vi "Neighbour Status.vi"(0 "Cell":i32, 5 "Parsed Board":T1, 11 "error in (no error)":errorcluster) -> (4 "Full?":bool, 6 "Min Count to Max":i32, 8 "Cell Index":i32, 15 "error out":errorcluster)   [LabVIEW 2014]
uses:
  Typedefs/Parsed Board.ctl
  Dragon Tamers.lvlib
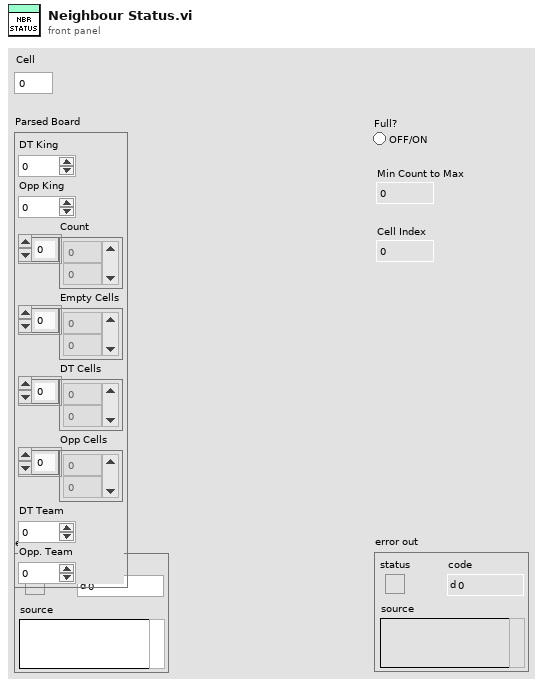
[diagram p1: front panel]
types:
  T1 = typedef "Dragon Tamers.lvlib/Parsed Board.ctl" = cluster{"DT King":i32, "Opp King":i32, "Count":i32[], "Empty Cells":i32[], "DT Cells":i32[], "Opp Cells":i32[], "DT Team":i32, "Opp. Team":i32}
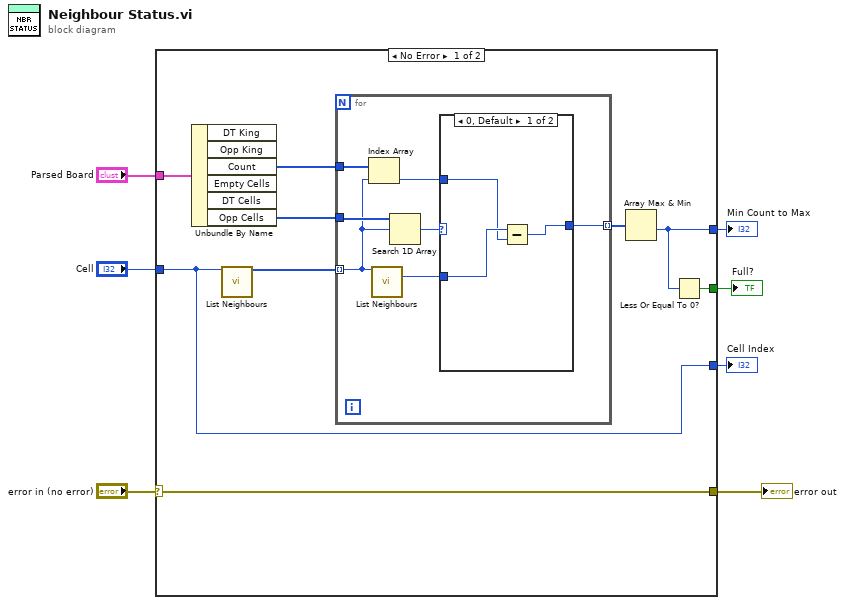
[diagram p0: block diagram]
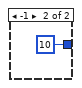
[diagram p2: hidden frame]
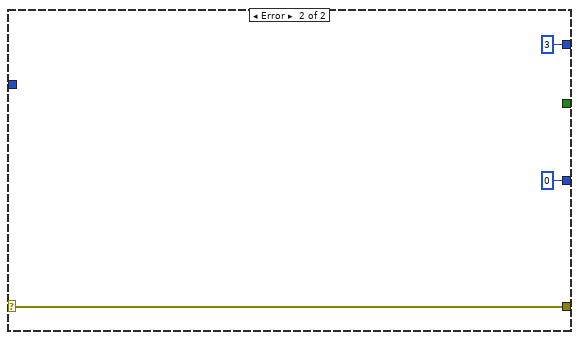
[diagram p3: hidden frame]
diagram:
  n1 = case shown="No Error" "error in (no error)" {
    selector: "error in (no error)" -> [w8 w30]
    tunnel: [w8 w30] -> w6
    tunnel: "Cell" -> [w9 _]
    tunnel: "Parsed Board" -> [w16 _]
    tunnel: [w12 3] -> w2
    tunnel: [w11 _] -> w3
    tunnel: [w9 0 ("Numeric")] -> w1
    frame No Error {
      n2 = Unbundle By Name(w16) -> ("Count"=w15:i32[], "Opp Cells"=w14:i32[])  [unwired: 4 out]
      n3 = call "List Neighbours.vi"("Cell Index"=w9) -> ("Neighbours"=w10:i32[])  [unwired: 12 in, 2 out]
      n4 = for {
        tunnel: w10 -> [w21] mode=indexing
        tunnel: w15 -> [w23]
        tunnel: w14 -> [w22]
        tunnel: [w17] -> w13 mode=indexing
        n5 = Index Array(array=w23, index=w21) -> (element=w19:i32)
        n6 = call "List Neighbours.vi"("Cell Index"=w21) -> ("Max Capacity"=w18:i32)  [unwired: 12 in, 2 out]
        n7 = Search 1D Array(1D array=w22, element=w21) -> (index of element=w20:i32)  [unwired: 1 in]
        n8 = case shown="0, Default" w20 {
          tunnel: w19 -> [w24 _]
          tunnel: w18 -> [w25 _]
          tunnel: [w26 10] -> w17
          frame 0, Default {
            n9 = Subtract(x=w25, y=w24) -> (x-y=w26:i32)
          }
          frame -1 {
          }
        }
      }
      n10 = Array Max & Min(array=w13) -> (min value=w12:i32)  [unwired: 3 out]
      n11 = Less Or Equal To 0?(x=w12) -> (x <= 0?=w11:bool)
    }
    frame Error {
    }
  }
  "error out" <- w6
  "Full?" <- w3
  "Min Count to Max" <- w2
  "Cell Index" <- w1
